vi "Set Stream Position.vi"(8 "error in (no error)":errorcluster, 10 "Read Position":i64, 11 "StringStream in":refnum<class "StringStream.lvclass">) -> (0 "error out":errorcluster, 3 "StringStream out":refnum<class "StringStream.lvclass">)   [LabVIEW 2020, in "Stream.lvlib" / "StringStream.lvclass"]
uses:
  StringStream.lvclass
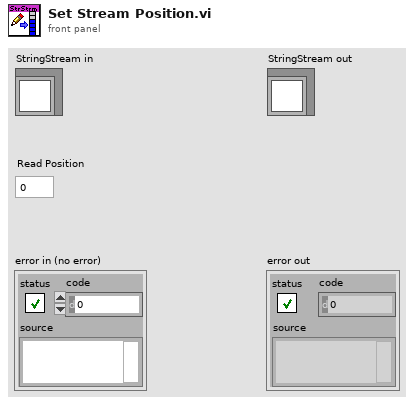
[diagram p1: front panel]
types:
  T1 = typedef "Stream.lvlib/StringStream.lvclass/Ref Data.ctl" = cluster{"Position":i64, "String":string}
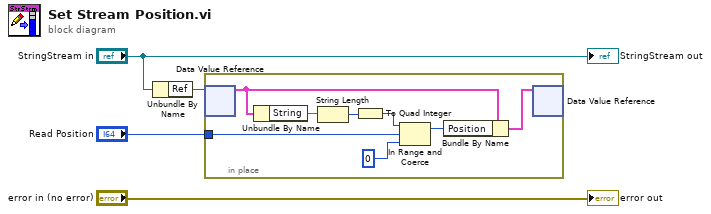
[diagram p0: block diagram]
diagram:
  n1 = Unbundle By Name("StringStream in") -> ("Ref"=w3:refnum<data-value>)
  n2 = in-place {
    in-place-border: "Read Position" -> [w7]
    n3 = in-place-dvr #1(w3) -> (w11:T1)  [unwired: 1 out]
    n4 = Unbundle By Name(w11) -> ("String"=w10:string)
    n5 = String Length(string=w10) -> (length=w9:i32)
    n6 = To Quad Integer(1:w9) -> (0:w5:i64)
    n7 = In Range and Coerce(upper limit=w5, x=w7, lower limit=i64 0) -> (coerced(x)=w6:i64)  [unwired: 1 out]
    n8 = Bundle By Name(cluster=w11, "Position"=w6) -> (w12:T1)
    n9 = in-place-dvr #1(w12) -> ()  [unwired: 2 out]
  }
  "error out" <- "error in (no error)"
  "StringStream out" <- "StringStream in"
